vi "Check External Triggers.vi"(8 "error in (no error)":errorcluster, 11 "Refs":T1 {"Channels" format="%.0x"; "Triggers" format="%.0x"}) -> (0 "error out":errorcluster, 3 "Refs":T1 {"Channels" format="%.0x"; "Triggers" format="%.0x"})   [LabVIEW 2020, in "Instrument Addon Engine.lvlib"]
uses:
  Instrument Addon Engine.lvlib
  Addon Shared/Types/External Trigger Refs.ctl
  <vilib>/NI VeriStand/Custom Device API/Data Reference.ctl
  <vilib>/NI VeriStand/Custom Device API/Global Data Refs.vi
  <vilib>/NI VeriStand/Custom Device API/Custom Device API.lvlib
  Addon Shared/Instrument Addon Shared.lvlib
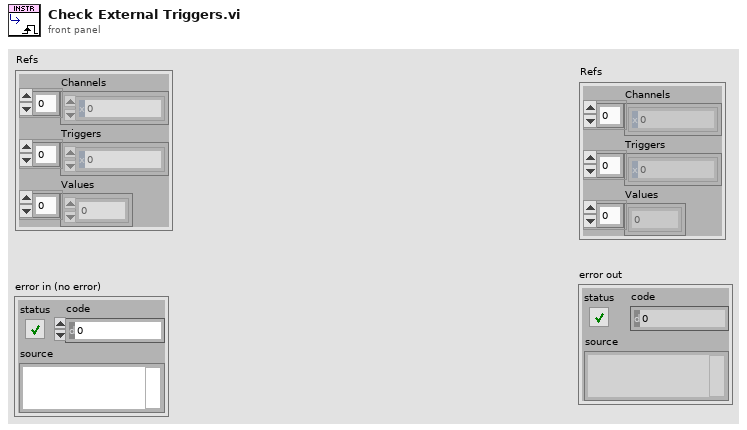
[diagram p1: front panel]
types:
  T1 = typedef "Instrument Addon Shared.lvlib/External Trigger Refs.ctl" = cluster{"Channels":T2[], "Triggers":T2[], "Values":dbl[]}
  T2 = typedef "Custom Device API.lvlib/Data Reference.ctl" = i32
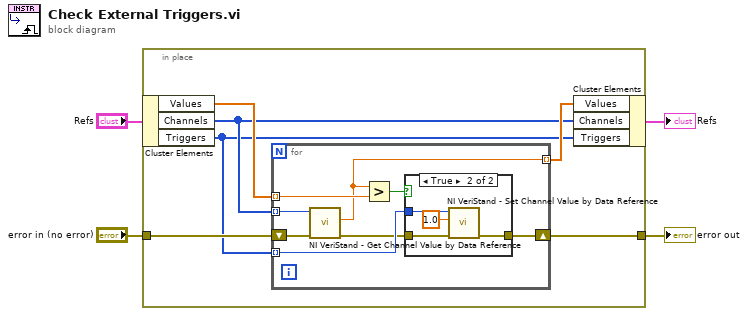
[diagram p0: block diagram]
diagram:
  n1 = in-place {
    in-place-border: [w8] -> w3
    in-place-border: "error in (no error)" -> [w7]
    n2 = in-place-cluster #1("Refs") -> ("Values"=w10:dbl[], "Channels"=w6:T2[], "Triggers"=w5:T2[])
    n3 = for {
      tunnel: w10 -> [w18] mode=indexing
      tunnel: [w17] -> w9 mode=indexing
      tunnel: w5 -> [w16] mode=indexing
      shift-right: [w13] -> w8
      shift-left: w7 -> [w12]
      tunnel: w6 -> [w11] mode=indexing
      n4 = call <vilib>:"NI VeriStand - Get Channel Value by Data Reference.vi"("error in (no error)"=w12, "Data Reference in"=w11) -> ("error out"=w14:errorcluster, "Value"=w17:dbl)  [unwired: 8 in]
      n5 = Greater?(x=w17, y=w18) -> (0:w15:bool)
      n6 = case shown="True" w15 {
        tunnel: w16 -> [_ w23]
        tunnel: w14 -> [w19 w21]
        tunnel: [w19 w20] -> w13
        frame False {
        }
        frame True {
          n7 = call <vilib>:"NI VeriStand - Set Channel Value by Data Reference.vi"("error in (no error)"=w21, "Value"=1.0, "Data Reference in"=w23) -> ("error out"=w20:errorcluster)  [unwired: 8 in]
        }
      }
    }
    n8 = in-place-cluster #1("Values"=w9, "Channels"=w6, "Triggers"=w5) -> (→"Refs":T1)
  }
  "error out" <- w3
